vi "Config SoftCal.vi"(0 "VISA resource name":refnum<visa-resource-name>, 1 "First Temp Point (4.2)":dbl=4.2 min=2.0 max=10.0 step=0.0001 format="%.4f", 2 "Scnd Temp Point (77.35)":dbl=77.35 min=50.0 max=100.0 step=0.0001 format="%.4f", 3 "Third Temp Point (305.0)":dbl=305.0 min=200.0 max=325.0 step=0.0001 format="%.4f", 5 "Standard Curve (0: DT-470)":u16(ring) items=["DT-470", "PT-100", "PT-1000"], 7 "User Curve (21)":dbl=21.0 min=21.0 max=28.0 step=1.0, 9 "Serial Number (0000)":string="000000", 11 "error in (no error)":errorcluster, 12 "First SensorPoint (1.62622)":dbl=1.62622 min=1.42039 max=1.6878 step=1e-05 format="%.5f", 13 "Second Sensor Point (1.02032)":dbl=1.02032 min=0.9755 max=1.07051 step=1e-05 format="%.5f", 14 "Third Sensor Point (0.50691)":dbl=0.50691 min=0.4586 max=0.75552 step=1e-05 format="%.5f") -> (4 "VISA resource name out":refnum<visa-resource-name>, 15 "error out":errorcluster)   [LabVIEW 2012, in "Lake Shore Cryotronics 218.lvlib"]
doc: "This VI enters the parameters to generate a softCal curve."
uses:
  <instrlib>/Lake Shore Cryotronics 218/Lake Shore Cryotronics 218.lvlib
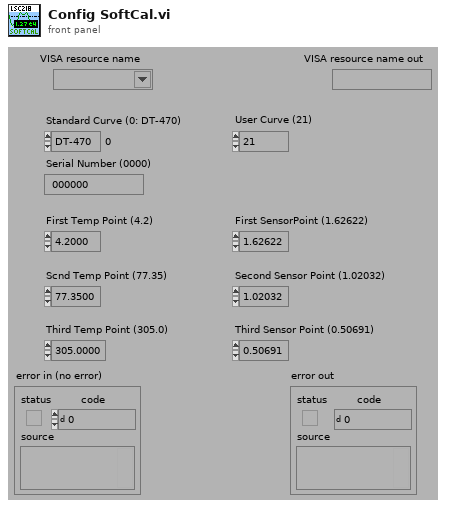
[diagram p1: front panel]
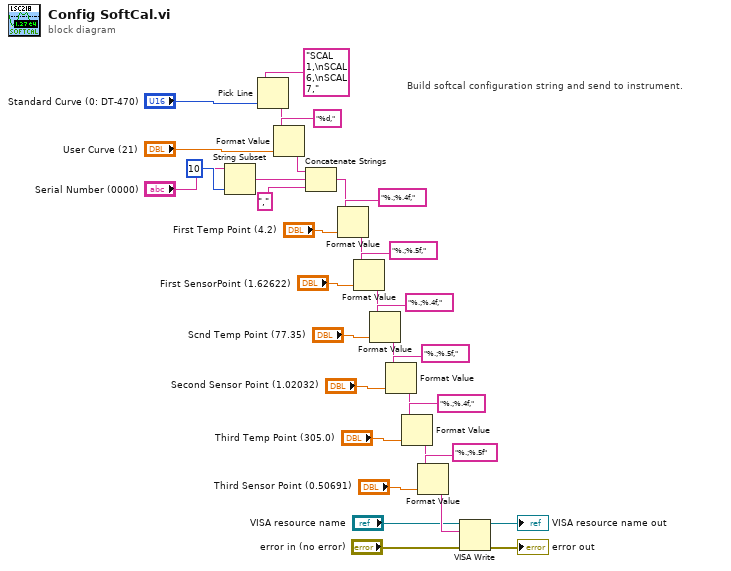
[diagram p0: block diagram]
diagram:
  # "Build softcal configuration string and send to instrument."
  n1 = String Subset(string="Serial Number (0000)", length (rest)=10) -> (substring=w32:string)  [unwired: 1 in]
  n2 = Pick Line(multi-line string="SCAL 1,\nSCAL 6,\nSCAL 7,", line index="Standard Curve (0: DT-470)") -> (output string=w5:string)  [unwired: 1 in]
  n3 = Format Value(string ("")=w5, format string="%d,", value (0)="User Curve (21)") -> (output string=w27:string)
  n4 = Concatenate Strings(w27, w32, ",") -> (w25:string)
  n5 = Format Value(string ("")=w25, format string="%.;%.4f,", value (0)="First Temp Point (4.2)") -> (output string=w8:string)
  n6 = Format Value(string ("")=w8, format string="%.;%.5f,", value (0)="First SensorPoint (1.62622)") -> (output string=w20:string)
  n7 = Format Value(string ("")=w20, format string="%.;%.4f,", value (0)="Scnd Temp Point (77.35)") -> (output string=w17:string)
  n8 = Format Value(string ("")=w17, format string="%.;%.5f,", value (0)="Second Sensor Point (1.02032)") -> (output string=w14:string)
  n9 = Format Value(string ("")=w14, format string="%.;%.4f,", value (0)="Third Temp Point (305.0)") -> (output string=w11:string)
  n10 = Format Value(string ("")=w11, format string="%.;%.5f", value (0)="Third Sensor Point (0.50691)") -> (output string=w9:string)
  n11 = VISA Write(VISA resource name="VISA resource name", write buffer=w9, error in (no error)="error in (no error)") -> (VISA resource name out=→"VISA resource name out":refnum<visa-resource-name>, error out=→"error out":errorcluster)  [unwired: 1 out]
